vi "CurrentInput_raw.vi"(8 "Mode":u16(ring) items=["Log w/ Exp Z", "Log w/ Lin Z"], 9 "Maximum (pA)":dbl=9000.0, 10 "Current (pA)":dbl format="%.1f", 11 "Setpoint (A)":dbl=100.0) -> (2 "Setpoint (pA)":dbl, 3 "Filtered Current (pA)":dbl format="%.1f", 7 "Safetip?":bool)   [LabVIEW 2019]
uses:
  <vilib>/Analysis/3filter.llb/Filter Passband Type.ctl
  <userlib>/HapticSTM/HapticSTM.lvlib
  <vilib>/ptbypt/NI_PtbyPt.lvlib
  <vilib>/Analysis/NI_AALBase.lvlib
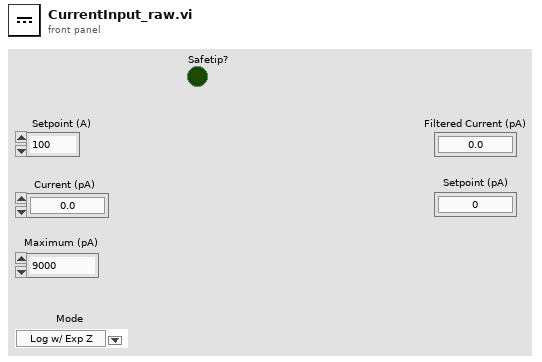
[diagram p1: front panel]
types:
  T1 = typedef "NI_AALBase.lvlib/Filter Passband Type.ctl" = enum32{"Lowpass", "Highpass", "Bandpass", "Bandstop"}
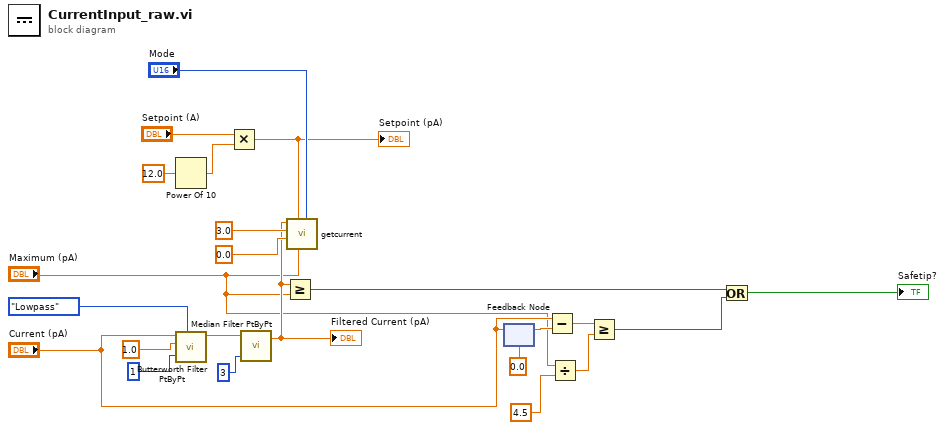
[diagram p0: block diagram]
diagram:
  n1 = Power Of 10(x=12.0) -> (10^x=w21:dbl)
  n2 = call <vilib>:"Butterworth Filter PtByPt.vi"("order"=1, "filter type"=Filter_Passband_Type."Lowpass", "sampling freq: fs"=1.0, "x"="Current (pA)") -> ("Filtered x"=w16:dbl)  [unwired: 5 in, 1 out]
  n3 = Multiply(x="Setpoint (A)", y=w21) -> (x*y=w12:dbl)
  "Setpoint (pA)" <- w12
  n4 = call <vilib>:"Median Filter PtByPt.vi"("rank"=3, "x"=w16) -> ("Filtered x"=w11:dbl)  [unwired: 2 in, 1 out]
  "Filtered Current (pA)" <- w11
  n5 = Greater Or Equal?(x=w11, y="Maximum (pA)") -> (x >= y?=w13:bool)
  n6 = call <userlib>:"getcurrent.vi"("forcemode"="Mode", "maxcurrentin"="Maximum (pA)", "setpoint"=w12, "minforcey"=0.0, "maxforcey"=3.0, "currentin"=w11) -> ()  [unwired: 6 in]
  n7 = feedback-in #1("Current (pA)") -> ()
  n8 = feedback #1(0.0 ("Current (pA)")) -> (w8:dbl)
  n9 = Subtract(x="Current (pA)", y=w8) -> (x-y=w5:dbl)
  n10 = Divide(x="Maximum (pA)", y=4.5) -> (x/y=w3:dbl)
  n11 = Greater Or Equal?(x=w5, y=w3) -> (x >= y?=w4:bool)
  n12 = Or(x=w13, y=w4) -> (x .or. y?=→"Safetip?":bool)
